vi "S_FILE_WRITER.VI"(2 "Data Write Format":enum16{"Real_Imag", "Mag_Angle", "dB_Angle"}(ring), 3 "error in (no error)":errorcluster, 4 "Data Input":T1={"Comments"="", "Ref Impedance"=75, "Trace Array"=[]} {"Trace Array"."Freq (Hz)" format="%.2e"; "Trace Array"."S-parameter Array" format="%.2f"}, 5 "Input Path":path) -> (0 "error out":errorcluster, 1 "Path After":path)   [LabVIEW 2017]
doc: "Writes data in Freq S Real Imag or Magnitude Angle \n9 Column Touchstone format \nfeatures write protection for existing files"
panel:
  # "Developed by :\nGregory Monahan & Art Morris \nDecember 1993"
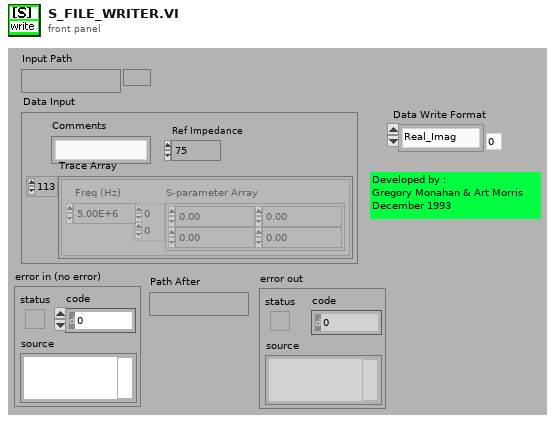
[diagram p1: front panel]
types:
  T1 = cluster{"Comments":string, "Ref Impedance":u16, "Trace Array":cluster{"Freq (Hz)":dbl, "S-parameter Array":csg[][]}[]}
  T2 = enum16{"open", "open or create", "create or replace", "create", "open (read only)"}
  T3 = cluster{"Freq (Hz)":dbl, "S-parameter Array":csg[][]}[]
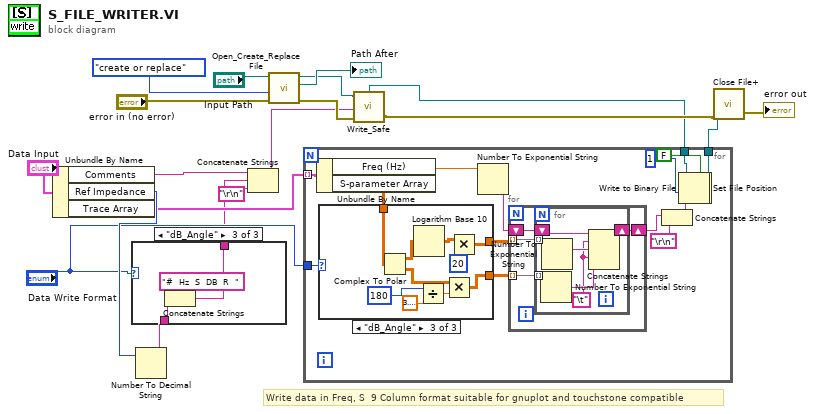
[diagram p0: block diagram]
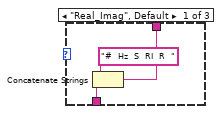
[diagram p2: hidden frame]
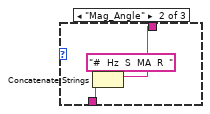
[diagram p3: hidden frame]
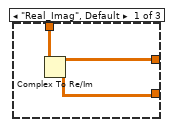
[diagram p4: hidden frame]
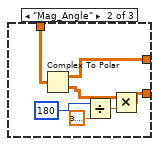
[diagram p5: hidden frame]
diagram:
  # "Write data in Freq, S  9 Column format suitable for gnuplot and touchstone compatible"
  n1 = Unbundle By Name("Data Input") -> ("Comments"=w8:string, "Ref Impedance"=w13:u16, "Trace Array"=w12:T3)
  n2 = Number To Decimal String(number=w13) -> (decimal integer string=w18:string)  [unwired: 1 out]
  n3 = case shown="\"dB_Angle\"" "Data Write Format" {
    tunnel: [w20 w23 w26] -> w7
    tunnel: w18 -> [w21 w25 w28]
    frame "Real_Imag", Default {
      n4 = Concatenate Strings("#  Hz  S  RI  R  ", w21) -> (w20:string)
    }
    frame "Mag_Angle" {
      n5 = Concatenate Strings("#  Hz  S  MA  R  ", w25) -> (w23:string)
    }
    frame "dB_Angle" {
      n6 = Concatenate Strings("#  Hz  S  DB  R  ", w28) -> (w26:string)
    }
  }
  n7 = Concatenate Strings(w8, w7, "\r\n") -> (w2:string)
  n8 = call <vilib>:"Open_Create_Replace File.vi"("error in (no error)"="error in (no error)", "function (open:0)"=T2."create or replace", "file path"="Input Path") -> ("error out"=w6:errorcluster, "new file path"=→"Path After":path, "refnum"=w3:refnum<file>)  [unwired: 3 in, 3 out]
  n9 = call "Write_Safe.vi"("error in"=w6, "Data"=w2, "refnum"=w3) -> ("error out"=w5:errorcluster, "dup refnum"=w4:refnum<file>)  [unwired: 1 out]
  n10 = for {
    tunnel: [w43] -> w19
    tunnel: w4 -> [w41]
    tunnel: w12 -> [w37] mode=indexing
    tunnel: "Data Write Format" -> [w32]
    n11 = Unbundle By Name(w37) -> ("Freq (Hz)"=w36:dbl, "S-parameter Array"=w35:csg[][])
    n12 = case shown="\"dB_Angle\"" w32 {
      tunnel: w35 -> [w47 w54 w64]
      tunnel: [w46 w53 w60] -> w34
      tunnel: [w45 w48 w55] -> w33
      frame "Real_Imag", Default {
        n13 = Complex To Re/Im(x + iy=w47) -> (x=w46:sgl[][], y=w45:sgl[][])
      }
      frame "Mag_Angle" {
        n14 = Complex To Polar(r * e^(i*theta)=w54) -> (r=w53:sgl[][], theta=w49:sgl[][])
        n15 = Divide(x=180, y=3.141592653589793) -> (x/y=w52:dbl)
        n16 = Multiply(x=w49, y=w52) -> (x*y=w48:dbl[][])
      }
      frame "dB_Angle" {
        n17 = Complex To Polar(r * e^(i*theta)=w64) -> (r=w63:sgl[][], theta=w57:sgl[][])
        n18 = Logarithm Base 10(1:w63) -> (0:w61:sgl[][])
        n19 = Divide(x=180, y=3.141592653589793) -> (x/y=w56:dbl)
        n20 = Multiply(x=w57, y=w56) -> (x*y=w55:dbl[][])
        n21 = Multiply(x=w61, y=20) -> (x*y=w60:sgl[][])
      }
    }
    n22 = Number To Exponential String(number=w36) -> (E-format string=w39:string)  [unwired: 3 out]
    n23 = for {
      shift-right: [w65] -> w38
      shift-left: w39 -> [w66]
      tunnel: w34 -> [w68] mode=indexing
      tunnel: w33 -> [w67] mode=indexing
      n24 = for {
        tunnel: w68 -> [w75] mode=indexing
        tunnel: w67 -> [w74] mode=indexing
        shift-right: [w70] -> w65
        shift-left: w66 -> [w69]
        w71 = "\t"
        n25 = Number To Exponential String(number=w74) -> (E-format string=w72:string)  [unwired: 3 out]
        n26 = Number To Exponential String(number=w75) -> (E-format string=w73:string)  [unwired: 3 out]
        n27 = Concatenate Strings(w69, w71, w73, w71, w72) -> (w70:string)
      }
    }
    n28 = Concatenate Strings(w38, "\r\n") -> (w44:string)
    n29 = Set File Position(refnum=w41, from (0:start)=1) -> (refnum out=w31:refnum<file>, error out=w30:errorcluster)  [unwired: 1 in, 1 out]
    n30 = Write to Binary File(file (use dialog)=w31, data=w44, error in=w30, 5:FALSE ("prepend array or string size? (T)")) -> (refnum out=w43:refnum<file>)  [unwired: 4 out]
  }
  n31 = call <vilib>:"Close File+.vi"("error in (no error)"=w5, "refnum"=w19) -> ("error out"=→"error out":errorcluster)  [unwired: 5 out]
